vi "set buffer.vi"(8 "error in (no error)":errorcluster, 11 "Thorcam in":refnum<class "Thorcam.lvclass">) -> (0 "error out":errorcluster, 3 "Thorcam out":refnum<class "Thorcam.lvclass">)   [LabVIEW 2012, in "Thorcam.lvclass"]
uses:
  Thorcam.lvclass
  Thorcam.lvclass/Thorcam.ctl
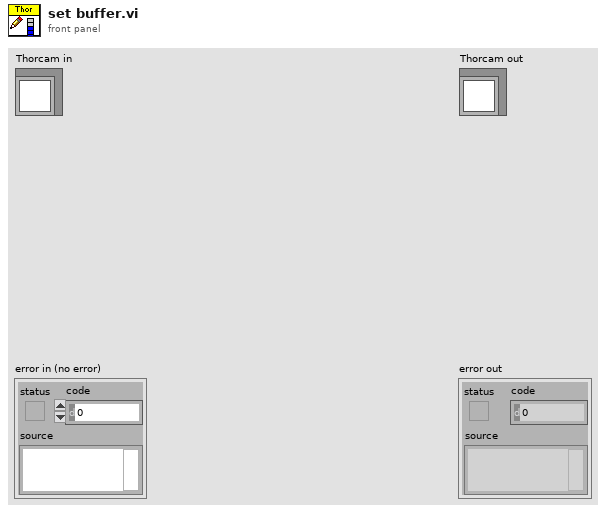
[diagram p1: front panel]
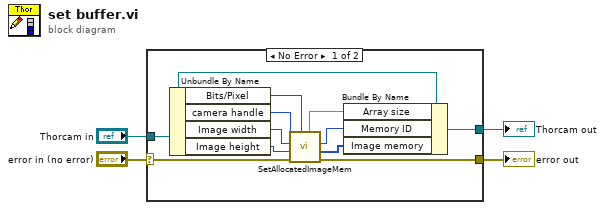
[diagram p0: block diagram]
diagram:
  n1 = case shown="No Error" "error in (no error)" {
    selector: "error in (no error)" -> [w14 w17]
    tunnel: [w6 w17] -> w3
    tunnel: [w5 w16] -> w1
    tunnel: "Thorcam in" -> [w10 w16]
    frame No Error {
      n2 = Unbundle By Name(w10) -> ("Bits/Pixel"=w11:i32, "camera handle"=w15:u32, "Image width"=w13:i32, "Image height"=w12:i32)
      n3 = call <instrlib>:"SetAllocatedImageMem.vi"("BitsPixel"=w11, "error in"=w14, "Height"=w12, "Width"=w13, "Camera Handle In"=w15) -> ("error out"=w6:errorcluster, "Image Memory Out"=w7:u8[], "Memory ID Out"=w8:i32, "Array Size"=w9:dbl)  [unwired: 2 in, 1 out]
      n4 = Bundle By Name(cluster=w10, "Array size"=w9, "Memory ID"=w8, "Image memory"=w7) -> (w5:refnum<class "Thorcam.lvclass">)
    }
    frame Error {
    }
  }
  "error out" <- w3
  "Thorcam out" <- w1
